vi "refgen.vi"(6 "Dynamic scaller: FBLR":dbl[](array[numeric]), 7 "Dynamic scaller: pry":dbl[](array[numeric]), 9 "Qube":refnum<class "System.lvclass">) -> (3 "Qube":refnum<class "System.lvclass">)   [LabVIEW 2021, in "System.lvclass"]
uses:
  System.lvclass
  System.lvclass/System.ctl
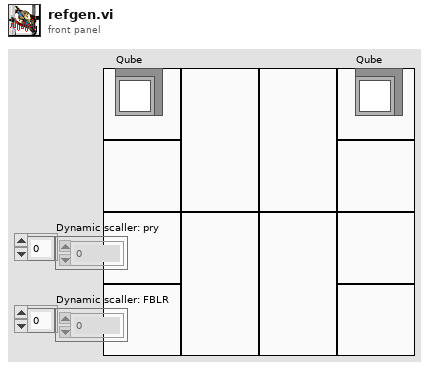
[diagram p1: front panel]
types:
  T1 = typedef "System.lvclass/mode.ctl" = enum16{"pry_OL", "pry_CL", "FBLR_CL"}
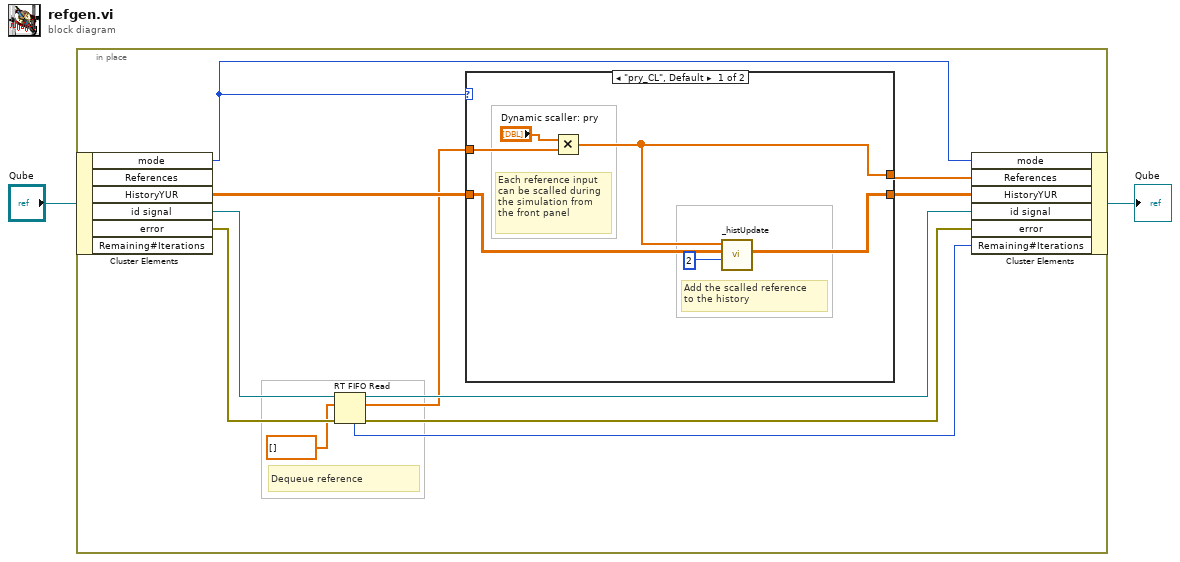
[diagram p0: block diagram]
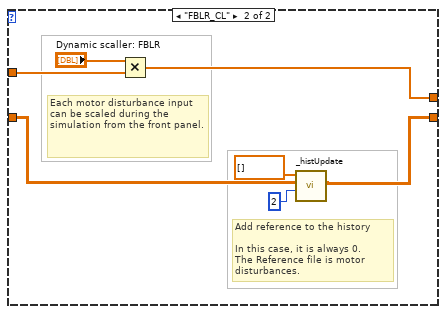
[diagram p2: hidden frame]
diagram:
  n1 = in-place {
    # "Dequeue reference"
    n2 = in-place-cluster #1("Qube") -> ("mode"=w4:T1, "HistoryYUR"=w8:dbl[][][], "id signal"=w10:refnum<k33>, "error"=w13:errorcluster)  [unwired: 2 out]
    n3 = RT FIFO Read(0:w10, 1:dbl[] [] ("element"), 3:w13) -> (7:w11:u32, 8:w5:refnum<k33>, 9:w3:dbl[], 11:w9:errorcluster)  [unwired: 1 in, 1 out]
    n4 = case shown="\"pry_CL\", Default" w4 {
      tunnel: w8 -> [w14 w21]
      tunnel: [w15 w23] -> w7
      tunnel: [w18 w20] -> w6
      tunnel: w3 -> [w19 w24]
      frame "pry_CL", Default {
        # "Each reference input\ncan be scalled during\nthe simulation from\nthe front panel"
        # "Add the scalled reference \nto the history"
        n5 = Multiply(x="Dynamic scaller: pry", y=w19) -> (x*y=w15:dbl[])
        n6 = call "_histUpdate.vi"("Y:0-U:1-R:2"=2, "History In"=w14, "pry"=w15) -> ("History Out"=w18:dbl[][][])  [unwired: 8 in]
      }
      frame "FBLR_CL" {
        # "Each motor disturbance input can be scaled during the simulation from the front panel."
        # "Add reference to the history\n\nIn this case, it is always 0. \nThe Reference file is motor \ndisturbances."
        n7 = Multiply(x="Dynamic scaller: FBLR", y=w24) -> (x*y=w23:dbl[])
        n8 = call "_histUpdate.vi"("Y:0-U:1-R:2"=2, "History In"=w21, "pry"=dbl[] [] ("Updating Array")) -> ("History Out"=w20:dbl[][][])  [unwired: 8 in]
      }
    }
    n9 = in-place-cluster #1("mode"=w4, "References"=w7, "HistoryYUR"=w6, "id signal"=w5, "error"=w9, "Remaining#Iterations"=w11) -> (→"Qube":refnum<class "System.lvclass">)
  }
